vi "DefineMulti1.vi"(6 "Label":string="Custom" caption="Label (\"Custom\")", 9 "Error in":errorcluster caption="Error in (no error)", 10 "Custom descriptions":string[](array[string]), 11 "Custom code":i32) -> ()   [LabVIEW 2017, in "GPError.lvlib"]
doc: "Dynamically defines a number of <B>Custom descriptions</B> for <B>Custom code</B> effective in this entire LabVIEW session. This custom code can later be set on the error wire as either an error or a warning from anywhere in the LabVIEW session by using the SetError or SetWarning functions.\n\nThe optional <B>Label</B> (default \"Custom\") will be common for all <B>Custom descriptions</B> and will be prepended each description like this: \"<Label>:\\s\\s<Description>\" to conform to the format of the built-in descriptions. Wire an empty string to <B>Label</B> to omit the label entirely from the description strings.\n\nIf you define a <B>Custom code</B> that has already been defined once, <B>Custom descriptions</B> will be appended to the existing array of descriptions for that <B>Custom code</B>. Any number of descriptions is supported for each code.\n\nIf you define descriptions for a <B>Custom code</B> that is a built-in error/warning code, then for the duration of this LabVIEW session these <B>Custom descriptions</B> for that code will be appended to the built-in description(s).\n\nAll defined descriptions for a <B>Custom code</B> can be deleted again dynamically with the UndefineCustomCode function.\n\nThis VI runs only if there is no error on <B>Error in</B>.\n\nThis VI is polymorphic, accepting either a single description or an array of descriptions to define.\n\nSteen Schmidt\nGPower\n17/7 2013"
uses:
  GPError.lvlib
panel:
  # "Copyright © 2013\nSteen Schmidt, GPower\nSee enclosed license file for terms and conditions"
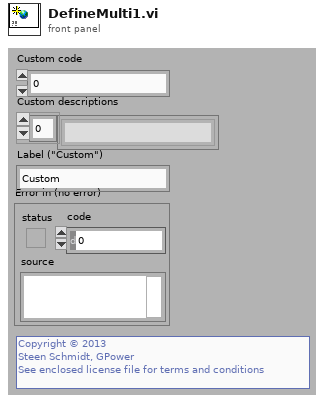
[diagram p1: front panel]
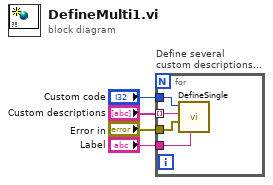
[diagram p0: block diagram]
diagram:
  n1 = for "Define several\ncustom descriptions..." {
    tunnel: "Custom descriptions" -> [w8] mode=indexing
    tunnel: "Label" -> [w7]
    tunnel: "Custom code" -> [w6]
    tunnel: "Error in" -> [w5]
    n2 = call "DefineSingle.vi"("Label"=w7, "Error in"=w5, "Custom description"=w8, "Custom code"=w6) -> ()  [unwired: 8 in]
  }
